vi "监测块.vi"(10 "索引":i32, 11 "数组":u16[](array[numeric])) -> (1 "string":string, 2 "数值":sgl, 3 "time stamp":timestamp)   [LabVIEW 2016, in "质控单元V1.lvlib"]
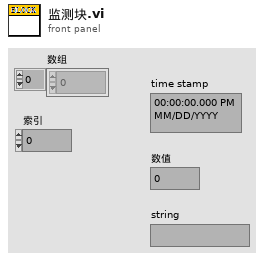
[diagram p1: front panel]
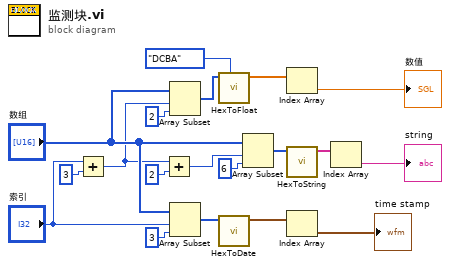
[diagram p0: block diagram]
diagram:
  n1 = Add(x="索引", y=3) -> (x+y=w4:i32)
  n2 = Add(x=w4, y=2) -> (x+y=w2:i32)
  n3 = Array Subset(array="数组", index=w4, length=2 ("长度")) -> (w13:u16[])
  n4 = Array Subset(array="数组", index="索引", length=3 ("长度")) -> (w8:u16[])
  n5 = call "HexToFloat.vi"("转换类型"=enum16{"DCBA", "CDAB"}."DCBA", "数组"=w13) -> ("FLOAT"=w14:sgl[])  [unwired: 9 in]
  n6 = call "HexToDate.vi"("数组"=w8) -> ("DATE"=w9:timestamp[])  [unwired: 10 in]
  n7 = Array Subset(array="数组", index=w2, length=6 ("长度")) -> (w17:u16[])
  n8 = Index Array(array=w14) -> (element=→"数值":sgl)  [unwired: 1 in]
  n9 = call "HexToString.vi"("数组"=w17) -> ("STRING"=w18:string[])  [unwired: 10 in]
  n10 = Index Array(array=w9) -> (element=→"time stamp":timestamp)  [unwired: 1 in]
  n11 = Index Array(array=w18) -> (element=→"string":string)  [unwired: 1 in]
